vi "Configure PID Loop Break Time.vi"(7 "Unit Address (1)":u8=1, 8 "error in (no error)":errorcluster, 10 "Loop Break Time (0)":i32, 11 "VISA resource name":refnum<visa-resource-name>) -> (0 "error out":errorcluster, 3 "VISA resource name out":refnum<visa-resource-name>)   [LabVIEW 2014, in "Eurotherm 35xx Series.lvlib"]
doc: "This VI sets PID Loop Break Time.\nThe loop break alarm may be disabled by setting its time to 0.\nThe loop break alarm attempts to detect loss of restoring action in the control loop by checking the control output, the process value and its rate of change.\nLoop break detection works for all control algorithms: PID, VP and ON-OFF.\n\nNote: This is not to be confused with load failure and partial load failure."
uses:
  <instrlib>/Eurotherm 35xx Series/Eurotherm 35xx Series.lvlib
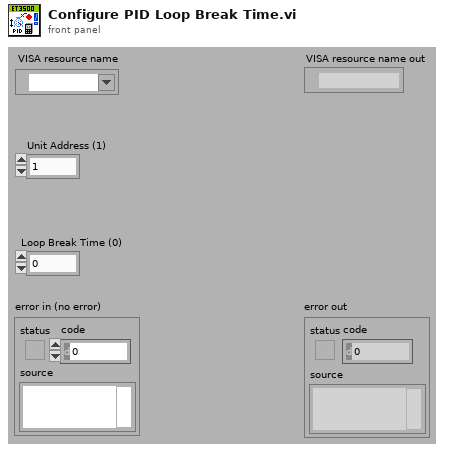
[diagram p1: front panel]
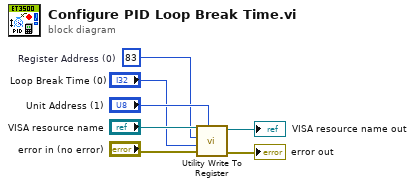
[diagram p0: block diagram]
diagram:
  w1 = 83  # Register Address (0)
  n1 = call <instrlib>:"Utility Write To Register.vi"("Unit Address (1)"="Unit Address (1)", "error in (no error)"="error in (no error)", "Data (0)"="Loop Break Time (0)", "Register Address (0)"=w1, "VISA resource name"="VISA resource name") -> ("error out"=→"error out":errorcluster, "VISA resource name out"=→"VISA resource name out":refnum<visa-resource-name>)  [unwired: 5 in]
